vi "Untitled 9.vi"() -> ()   [LabVIEW 2024]
panel:
  out "result string":string
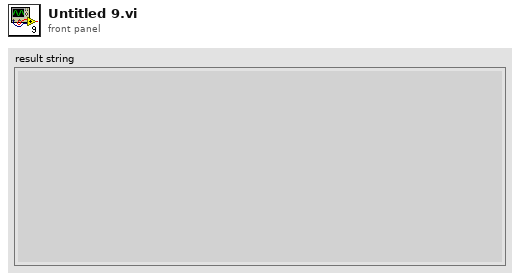
[diagram p1: front panel]
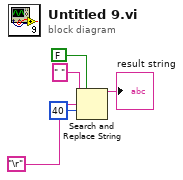
[diagram p0: block diagram]
diagram:
  n1 = Search and Replace String(replace all?=FALSE ("replace all? (F)"), search string=" ", replace string="\r", offset=40 ("offset (0)")) -> (result string=→"result string":string)  [unwired: 4 in, 3 out]
